vi "F8588A Initialize Digitizing Mode.vi"(4 "Ext Guard (false)":bool, 5 "dmm 8588 pll (off)":T2 caption="Fluke 8588A phase lock (off)", 6 "Low Pass Filter (off)":T3 caption="Fluke 8588A Low Pass", 7 "range [V] (10V)":dbl=10.0, 8 "error in (no error)":errorcluster, 9 "dmm couple (DC auto)":T1=enum."DC, auto", 10 "Reset (True)":bool, 11 "VISA DMM":refnum<visa-resource-name>) -> (0 "error out":errorcluster, 1 "sample memory [B]":i32, 2 "idn string":string, 3 "VISA resource name out":refnum<visa-resource-name>)   [LabVIEW 2020]
doc: "This VI does basic configuration of DMM for digitizing. It stops sampling, exports sync pulses to EXTOUT and does few more global settings that don't need to be changed for the measurement itself.\n\nNote: Reentrant VI so it can be executed in parallel for multiple DMM sessions."
uses:
  F8588A Low Pass Filter.ctl
  F8588A Phase Lock.ctl
  F8588A Coupling.ctl
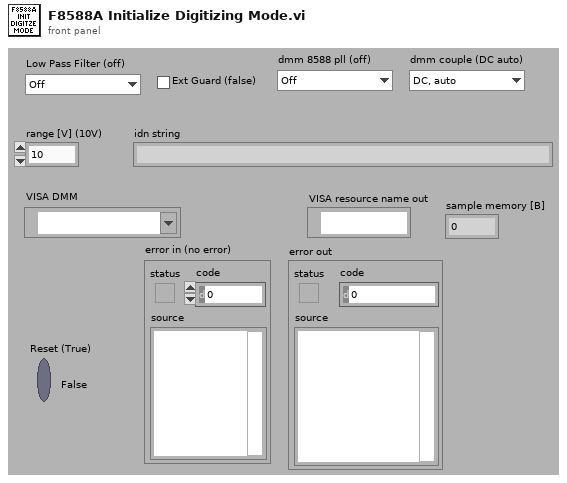
[diagram p1: front panel]
types:
  T1 = typedef "F8588A Coupling.ctl" = enum16{"AC, 1 MOhm", "AC, 10 MOhm", "DC, 1 MOhm", "DC, 10 MOhm", "DC, auto"}
  T2 = typedef "F8588A Phase Lock.ctl" = enum16{"Off", "1 MHz", "10 MHz"}
  T3 = typedef "F8588A Low Pass Filter.ctl" = enum16{"Off", "100 kHz", "3 MHz"}
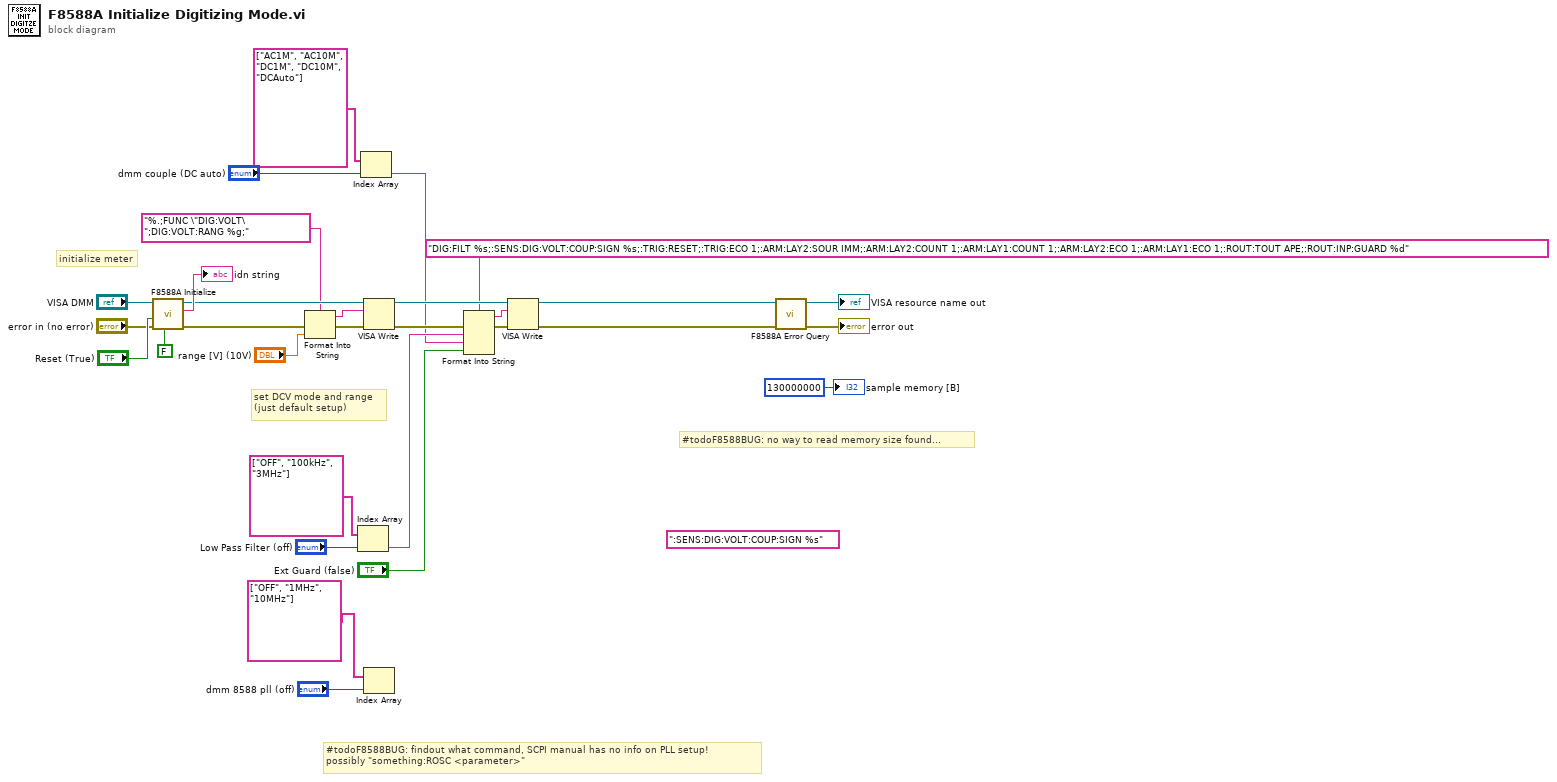
[diagram p0: block diagram]
diagram:
  (unwired) ":SENS:DIG:VOLT:COUP:SIGN %s" ("write buffer")
  # "#todoF8588BUG: findout what command, SCPI manual has no info on PLL setup!\npossibly \"something:ROSC <parameter>\""
  # "#todoF8588BUG: no way to read memory size found..."
  # "set DCV mode and range\n(just default setup)"
  # "initialize meter"
  n1 = call "F8588A Initialize.vi"("Allow go to default? (True)"=FALSE ("Allow go to default? (False)"), "error in (no error)"="error in (no error)", "Reset (True)"="Reset (True)", "VISA resource name"="VISA DMM") -> ("error out"=w23:errorcluster, "idn string"=→"idn string":string, "VISA resource name out"=w22:refnum<visa-resource-name>)  [unwired: 5 in]
  n2 = Format Into String(format string="%.;FUNC \"DIG:VOLT\";DIG:VOLT:RANG %g;" ("write buffer"), error in=w23, "range [V] (10V)") -> (resulting string=w17:string, error out=w26:errorcluster)  [unwired: 1 in]
  n3 = Index Array(array=string[] ["OFF", "100kHz", "3MHz"], index="Low Pass Filter (off)") -> (element=w8:string)
  n4 = Index Array(array=string[] ["AC1M", "AC10M", "DC1M", "DC10M", "DCAuto"], index="dmm couple (DC auto)") -> (element=w1:string)
  n5 = VISA Write(VISA resource name=w22, write buffer=w17, error in (no error)=w26) -> (VISA resource name out=w24:refnum<visa-resource-name>, error out=w7:errorcluster)  [unwired: 1 out]
  n6 = Index Array(array=string[] ["OFF", "1MHz", "10MHz"], index="dmm 8588 pll (off)") -> ()  [unwired: 1 out]
  n7 = Format Into String(format string="DIG:FILT %s;:SENS:DIG:VOLT:COUP:SIGN %s;:TRIG:RESET;:TRIG:ECO 1;:ARM:LAY2:SOUR IMM;:ARM:LAY2:COUNT 1;:ARM:LAY1:COUNT 1;:ARM:LAY2:ECO 1;:ARM:LAY1:ECO 1;:ROUT:TOUT APE;:ROUT:INP:GUARD %d" ("write buffer"), error in=w7, w8, w1, "Ext Guard (false)") -> (resulting string=w12:string, error out=w13:errorcluster)  [unwired: 1 in]
  n8 = VISA Write(VISA resource name=w24, write buffer=w12, error in (no error)=w13) -> (VISA resource name out=w14:refnum<visa-resource-name>, error out=w15:errorcluster)  [unwired: 1 out]
  n9 = call "F8588A Error Query.vi"("error in (no error)"=w15, "VISA resource name"=w14) -> ("error out"=→"error out":errorcluster, "VISA resource name out"=→"VISA resource name out":refnum<visa-resource-name>)  [unwired: 6 in, 2 out]
  "sample memory [B]" <- 130000000 ("sample memory [B]")
